vi "Configure Timer (Relative).vi"(0 "VISA resource name":refnum<visa-resource-name>, 1 "Interval Day (0)":i32 min=0 max=31, 2 "Interval Hour (1)":i32=1 min=0 max=23, 3 "Interval Minute (0)":i32 min=0 max=59, 5 "Timer No. (1)":i32=1 min=1 max=12, 7 "Reset (True)":bool=TRUE, 11 "error in (no error)":errorcluster) -> (4 "VISA resource name out":refnum<visa-resource-name>, 6 "Timer No.":i32, 15 "error out":errorcluster)   [LabVIEW 2020, in "Yokogawa GX Series.lvlib"]
doc: "Sets a Relative timer.\n\nCommand: STimer"
uses:
  <instrlib>/Yokogawa GX Series/Yokogawa GX Series.lvlib
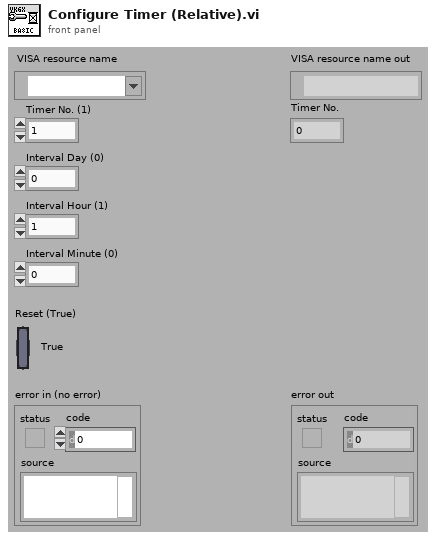
[diagram p1: front panel]
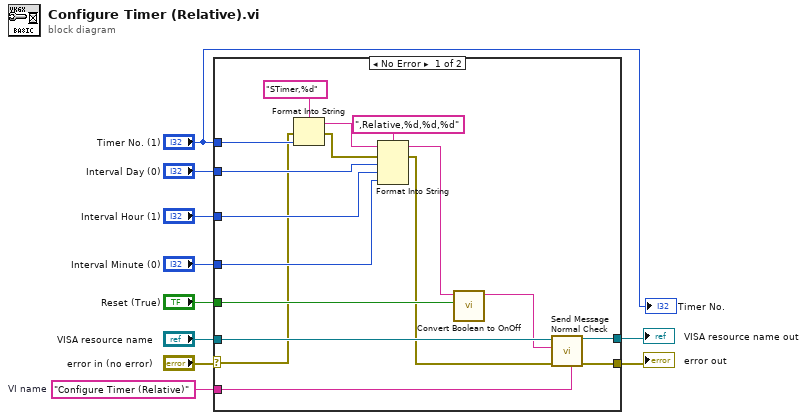
[diagram p0: block diagram]
diagram:
  w10 = "Configure Timer (Relative)"  # VI name
  n1 = case shown="No Error" "error in (no error)" {
    selector: "error in (no error)" -> [w11 w28]
    tunnel: w10 -> [w27 _]
    tunnel: [w26 w29] -> w1
    tunnel: [w25 w28] -> w9
    tunnel: "VISA resource name" -> [w22 w29]
    tunnel: "Interval Day (0)" -> [w21 _]
    tunnel: "Interval Hour (1)" -> [w20 _]
    tunnel: "Interval Minute (0)" -> [w19 _]
    tunnel: "Reset (True)" -> [w18 _]
    tunnel: "Timer No. (1)" -> [w12 _]
    frame No Error {
      n2 = Format Into String(format string="STimer,%d", error in=w11, w12) -> (resulting string=w23:string, error out=w17:errorcluster)  [unwired: 1 in]
      n3 = Format Into String(format string=",Relative,%d,%d,%d", initial string=w23, error in=w17, w21, w20, w19) -> (resulting string=w14:string, error out=w16:errorcluster)
      n4 = call <instrlib>:"Convert Boolean to OnOff.vi"("On/Off"=w18, "Initial String (\"\")"=w14) -> ("Resulting String"=w13:string)  [unwired: 9 in]
      n5 = call <instrlib>:"Send Message Normal Check.vi"("Source (\"\")"=w27, "error in (no error)"=w16, "Send Message (\"\")"=w13, "VISA resource name"=w22) -> ("error out"=w25:errorcluster, "VISA resource name out"=w26:refnum<visa-resource-name>)  [unwired: 2 in, 4 out]
    }
    frame Error {
    }
  }
  "error out" <- w9
  "VISA resource name out" <- w1
  "Timer No." <- "Timer No. (1)"
